vi "constructEnumerationControl.vi"(8 "error in (no error)":errorcluster, 10 "libraryInfo":T1, 11 "Enumeration in":refnum<class "Enumeration.lvclass">) -> (0 "error out":errorcluster, 3 "Enumeration out":refnum<class "Enumeration.lvclass">)   [LabVIEW 2018, in "Enumeration.lvclass"]
uses:
  Enumeration.lvclass
  Typedefs/LibraryInfo.ctl
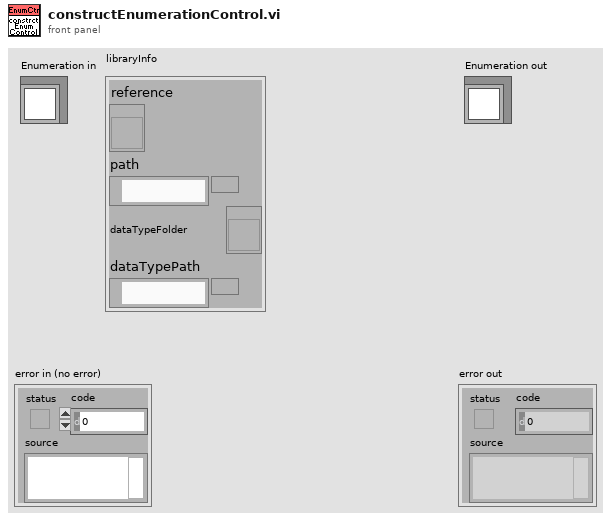
[diagram p1: front panel]
types:
  T1 = typedef "LibraryInfo.ctl" = cluster{"reference":refnum<vi>, "path":path, "dataTypeFolder":refnum<vi>, "dataTypePath":path}
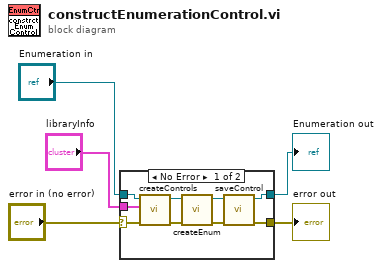
[diagram p0: block diagram]
diagram:
  n1 = case shown="No Error" "error in (no error)" {
    selector: "error in (no error)" -> [w12 w16]
    tunnel: [w10 w16] -> w4
    tunnel: [w11 w15] -> w2
    tunnel: "Enumeration in" -> [w14 w15]
    tunnel: "libraryInfo" -> [w13 _]
    frame No Error {
      n2 = call "createControls.vi"("error in (no error)"=w12, "libraryInfo"=w13, "Enumeration in"=w14) -> ("error out"=w6:errorcluster, "Enumeration out"=w9:refnum<class "Enumeration.lvclass">)  [unwired: 7 in]
      n3 = call "createEnum.vi"("error in (no error)"=w6, "Enumeration in"=w9) -> ("error out"=w7:errorcluster, "Enumeration out"=w8:refnum<class "Enumeration.lvclass">)  [unwired: 8 in]
      n4 = call "saveControl.vi"("error in (no error)"=w7, "Enumeration in"=w8) -> ("error out"=w10:errorcluster, "Enumeration out"=w11:refnum<class "Enumeration.lvclass">)  [unwired: 8 in]
    }
    frame Error {
    }
  }
  "error out" <- w4
  "Enumeration out" <- w2
